vi "151126 thruster.vi"() -> ()   [LabVIEW 2015]
uses:
  <vilib>/MakerHub/LINX/Private/Type Defs/User Platform.ctl
  <vilib>/MakerHub/LINX/Private/Device/Type Defs/TCP Config.ctl
  <vilib>/MakerHub/LINX/Private/Type Defs/Interface.ctl
  <vilib>/MakerHub/LINX/Public/Sensors/Motion/Servo/Servo Open One Channel.vi
  <vilib>/MakerHub/Xbox-One-Controller/Public/Open First Controller.vi
  <vilib>/MakerHub/LINX/Public/Sensors/Motion/Servo/Servo Set Pulse Width One Channel.vi
  <vilib>/MakerHub/LINX/Public/Sensors/Motion/Servo/Servo Close One Channel.vi
  <vilib>/MakerHub/Xbox-One-Controller/LMH-Xbox-One-Controller.lvlib
  <vilib>/MakerHub/LINX/LMH-LINX.lvlib
  <vilib>/MakerHub/LINX/Public/Sensors/Motion/Servo/Servo.lvlib
  <vilib>/MakerHub/LINX/Private/Device/Device.lvlib
panel:
  in  "Stop Button":bool
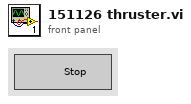
[diagram p1: front panel]
types:
  T1 = typedef "LMH-LINX.lvlib/Interface.ctl" = enum16{"Serial", "TCP"}
  T2 = typedef "LMH-LINX.lvlib/Device.lvlib/TCP Config.ctl" = cluster{"IP Address":string, "Port":u16}
  T3 = typedef "LMH-LINX.lvlib/User Platform.ctl" = enum16{"Default", "LINX", "myRIO"}
  T4 = typedef "LMH-LINX.lvlib/LINX Ref.ctl" = cluster{"Platform":T5, "Interface":T1, "LINX Device Config":T6}
  T5 = typedef "LMH-LINX.lvlib/Platform.ctl" = enum16{"LINX", "myRIO"}
  T6 = typedef "LMH-LINX.lvlib/Device.lvlib/LINX Device Config.ctl" = cluster{"Interface":T1, "COM Port":refnum<visa-resource-name>, "TCP Configuration":T2, "Device Family":u8, "Device ID":u8, "Device Name":string, "TCP Ref":refnum<k5>, "Channels":T7}
  T7 = typedef "LMH-LINX.lvlib/Channels.ctl" = cluster{"DI":u8[], "DO":u8[], "AI":u8[], "AO":u8[], "PWM":u8[], "QE":u8[], "UART":u8[], "I2C 2":u8[], "SPI":u8[], "CAN":u8[], "Servo":u8[], "AI Ref (V)":dbl, "AO Ref (V)":dbl, "AO Resolution (Bits)":u8}
  T8 = typedef "LMH-Xbox-One-Controller.lvlib/Xbox One Controller Ref.ctl" = cluster{"Controller Ref":refnum<k1>, "Event Refnum":refnum<event-registration>, "Worker Ref":refnum<vi>}
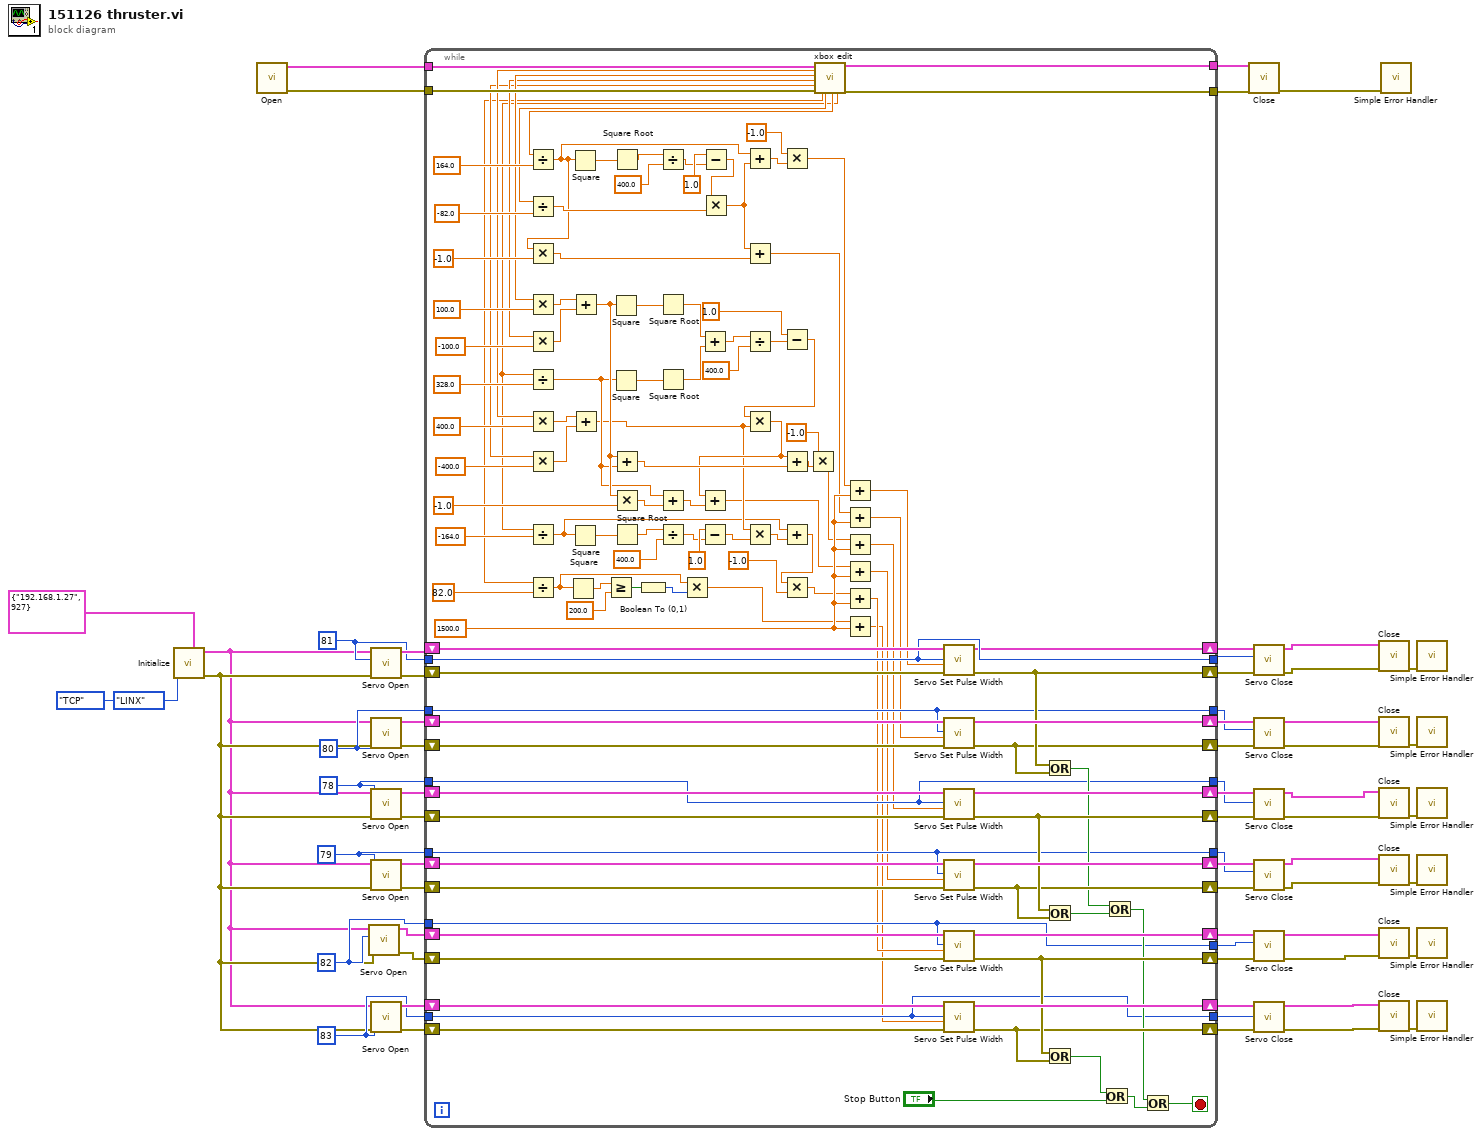
[diagram p0: block diagram]
diagram:
  w34 = u8 83 ("Servo Channel 6")
  w22 = u8 82 ("Servo Channel 5")
  w33 = u8 79 ("Servo Channel 4")
  w32 = u8 78 ("Servo Channel 3")
  w31 = u8 80 ("Servo Channel 2")
  w30 = u8 81 ("Servo Channel")
  n1 = call <vilib>:"Initialize.vi"("TCP Configuration"=T2 {"IP Address"="192.168.1.27", "Port"=927}, "Interface"=Interface."TCP", "Platform"=User_Platform."LINX") -> ("Error Out"=w3:errorcluster, "LINX Ref"=w2:T4)  [unwired: 6 in, 1 out]
  n2 = call-poly <vilib>:"Open.vi"() -> ("Error Out"=w36:errorcluster, "Xbox One Controller"=w38:T8)  [unwired: 9 in, 1 out]
  n3 = call-poly <vilib>:"Servo Open.vi"("Error In"=w3, "Servo Channel"=w22, "LINX Resource"=w2) -> ("Error Out"=w23:errorcluster, "LINX Resource"=w24:T4)  [unwired: 7 in]
  n4 = call-poly <vilib>:"Servo Open.vi"("Error In"=w3, "Servo Channel"=w30, "LINX Resource"=w2) -> ("Error Out"=w63:errorcluster, "LINX Resource"=w58:T4)  [unwired: 7 in]
  n5 = call-poly <vilib>:"Servo Open.vi"("Error In"=w3, "Servo Channel"=w31, "LINX Resource"=w2) -> ("Error Out"=w62:errorcluster, "LINX Resource"=w57:T4)  [unwired: 7 in]
  n6 = call-poly <vilib>:"Servo Open.vi"("Error In"=w3, "Servo Channel"=w32, "LINX Resource"=w2) -> ("Error Out"=w61:errorcluster, "LINX Resource"=w56:T4)  [unwired: 7 in]
  n7 = call-poly <vilib>:"Servo Open.vi"("Error In"=w3, "Servo Channel"=w33, "LINX Resource"=w2) -> ("Error Out"=w60:errorcluster, "LINX Resource"=w55:T4)  [unwired: 7 in]
  n8 = call-poly <vilib>:"Servo Open.vi"("Error In"=w3, "Servo Channel"=w34, "LINX Resource"=w2) -> ("Error Out"=w59:errorcluster, "LINX Resource"=w54:T4)  [unwired: 7 in]
  n9 = while {
    shift-right: [w66] -> w50
    shift-left: w58 -> [w180]
    shift-right: [w169] -> w44
    shift-left: w63 -> [w186]
    shift-right: [w174] -> w49
    shift-left: w57 -> [w179]
    shift-right: [w168] -> w43
    shift-left: w62 -> [w185]
    shift-right: [w173] -> w48
    shift-left: w56 -> [w178]
    shift-right: [w167] -> w42
    shift-left: w61 -> [w184]
    shift-right: [w172] -> w47
    shift-left: w55 -> [w177]
    shift-right: [w166] -> w41
    shift-left: w60 -> [w183]
    shift-right: [w171] -> w46
    shift-left: w24 -> [w176]
    shift-right: [w165] -> w40
    shift-left: w23 -> [w182]
    shift-right: [w170] -> w45
    shift-left: w54 -> [w175]
    shift-right: [w164] -> w39
    shift-left: w59 -> [w181]
    tunnel: w38 -> [w158]
    tunnel: [w157] -> w37
    tunnel: w36 -> [w156]
    tunnel: [w155] -> w35
    tunnel: w34 -> [w149]
    tunnel: w22 -> [w150]
    tunnel: w33 -> [w151]
    tunnel: w32 -> [w152]
    tunnel: w31 -> [w153]
    tunnel: w30 -> [w154]
    tunnel: [w154] -> w1
    tunnel: [w153] -> w29
    tunnel: [w152] -> w28
    tunnel: [w151] -> w27
    tunnel: [w150] -> w26
    tunnel: [w149] -> w25
    stop <- w65 stop-if-true
    w148 = 1500.0
    n10 = call "xbox edit.vi"("Xbox One Controller Ref"=w158, "Error In"=w156) -> ("Y"=w108:dbl, "B"=w125:dbl, "X"=w124:dbl, "A 2"=w107:dbl, "LS X"=w84:dbl, "LS Y"=w132:dbl, "RS X"=w142:dbl, "RS Y"=w79:dbl, "Xbox One Controller Ref"=w157:T8, "Error Out"=w155:errorcluster)  [unwired: 8 in]
    n11 = Divide(x=w142, y=164.0) -> (x/y=w131:dbl)
    n12 = Divide(x=w132, y=-82.0) -> (x/y=w140:dbl)
    n13 = Multiply(x=w131, y=-1.0) -> (x*y=w130:dbl)
    n14 = Multiply(x=w125, y=100.0) -> (x*y=w123:dbl)
    n15 = Multiply(x=w124, y=-100.0) -> (x*y=w122:dbl)
    n16 = Divide(x=w79, y=328.0) -> (x/y=w102:dbl)
    n17 = Multiply(x=w108, y=400.0) -> (x*y=w112:dbl)
    n18 = Multiply(x=w107, y=-400.0) -> (x*y=w111:dbl)
    n19 = Divide(x=w79, y=-164.0) -> (x/y=w88:dbl)
    n20 = Divide(x=w84, y=82.0) -> (x/y=w81:dbl)
    n21 = Square(x=w81) -> (x^2=w83:dbl)
    n22 = Square(x=w131) -> (x^2=w139:dbl)
    n23 = Square(x=w88) -> (x^2=w97:dbl)
    n24 = Add(x=w123, y=w122) -> (x+y=w103:dbl)
    n25 = Add(x=w112, y=w111) -> (x+y=w91:dbl)
    n26 = Greater Or Equal?(x=w83, y=200.0) -> (x >= y?=w87:bool)
    n27 = Square(x=w103) -> (x^2=w120:dbl)
    n28 = Square(x=w102) -> (x^2=w119:dbl)
    n29 = Square Root(x=w139) -> (sqrt(x)=w138:dbl)
    n30 = Add(x=w103, y=w102) -> (x+y=w105:dbl)
    n31 = Multiply(x=w103, y=-1.0) -> (x*y=w101:dbl)
    n32 = Square Root(x=w97) -> (sqrt(x)=w96:dbl)
    n33 = Boolean To (0,1)(Boolean=w87) -> (0, 1=w86:i16)
    n34 = Divide(x=w138, y=400.0) -> (x/y=w135:dbl)
    n35 = Square Root(x=w120) -> (sqrt(x)=w117:dbl)
    n36 = Square Root(x=w119) -> (sqrt(x)=w118:dbl)
    n37 = Add(x=w102, y=w101) -> (x+y=w100:dbl)
    n38 = Divide(x=w96, y=400.0) -> (x/y=w93:dbl)
    n39 = Multiply(x=w81, y=w86) -> (x*y=w80:dbl)
    n40 = Add(x=w117, y=w118) -> (x+y=w116:dbl)
    n41 = Subtract(x=1.0, y=w93) -> (x-y=w92:dbl)
    n42 = Subtract(x=1.0, y=w135) -> (x-y=w134:dbl)
    n43 = Multiply(x=w134, y=w140) -> (x*y=w129:dbl)
    n44 = Add(x=w131, y=w129) -> (x+y=w76:dbl)
    n45 = Add(x=w129, y=w130) -> (x+y=w128:dbl)
    n46 = Divide(x=w116, y=400.0) -> (x/y=w114:dbl)
    n47 = Multiply(x=w91, y=w92) -> (x*y=w89:dbl)
    n48 = Multiply(x=-1.0, y=w76) -> (x*y=w74:dbl)
    n49 = Subtract(x=1.0, y=w114) -> (x-y=w106:dbl)
    n50 = Multiply(x=w106, y=w91) -> (x*y=w99:dbl)
    n51 = Add(x=w99, y=w100) -> (x+y=w90:dbl)
    n52 = Add(x=w99, y=w105) -> (x+y=w73:dbl)
    n53 = Add(x=w88, y=w89) -> (x+y=w70:dbl)
    n54 = Multiply(x=w70, y=-1.0) -> (x*y=w68:dbl)
    n55 = Multiply(x=-1.0, y=w73) -> (x*y=w71:dbl)
    n56 = Add(x=w74, y=w148) -> (x+y=w144:dbl)
    n57 = Add(x=w128, y=w148) -> (x+y=w145:dbl)
    n58 = Add(x=w71, y=w148) -> (x+y=w146:dbl)
    n59 = Add(x=w90, y=w148) -> (x+y=w147:dbl)
    n60 = Add(x=w68, y=w148) -> (x+y=w78:dbl)
    n61 = Add(x=w80, y=w148) -> (x+y=w77:dbl)
    n62 = call-poly <vilib>:"Servo Set Pulse Width.vi"("Error In"=w186, "Pulse Width (uS)"=w144, "Servo Channel"=w154, "LINX Resource"=w180) -> ("Error Out"=w169:errorcluster, "LINX Resource"=w66:T4)  [unwired: 6 in]
    n63 = call-poly <vilib>:"Servo Set Pulse Width.vi"("Error In"=w185, "Pulse Width (uS)"=w145, "Servo Channel"=w153, "LINX Resource"=w179) -> ("Error Out"=w168:errorcluster, "LINX Resource"=w174:T4)  [unwired: 6 in]
    n64 = call-poly <vilib>:"Servo Set Pulse Width.vi"("Error In"=w184, "Pulse Width (uS)"=w146, "Servo Channel"=w152, "LINX Resource"=w178) -> ("Error Out"=w167:errorcluster, "LINX Resource"=w173:T4)  [unwired: 6 in]
    n65 = call-poly <vilib>:"Servo Set Pulse Width.vi"("Error In"=w183, "Pulse Width (uS)"=w147, "Servo Channel"=w151, "LINX Resource"=w177) -> ("Error Out"=w166:errorcluster, "LINX Resource"=w172:T4)  [unwired: 6 in]
    n66 = call-poly <vilib>:"Servo Set Pulse Width.vi"("Error In"=w182, "Pulse Width (uS)"=w78, "Servo Channel"=w150, "LINX Resource"=w176) -> ("Error Out"=w165:errorcluster, "LINX Resource"=w171:T4)  [unwired: 6 in]
    n67 = call-poly <vilib>:"Servo Set Pulse Width.vi"("Error In"=w181, "Pulse Width (uS)"=w77, "Servo Channel"=w149, "LINX Resource"=w175) -> ("Error Out"=w164:errorcluster, "LINX Resource"=w170:T4)  [unwired: 6 in]
    n68 = Or(x=w169, y=w168) -> (x .or. y?=w162:bool)
    n69 = Or(x=w167, y=w166) -> (x .or. y?=w163:bool)
    n70 = Or(x=w165, y=w164) -> (x .or. y?=w161:bool)
    n71 = Or(x=w161, y="Stop Button") -> (x .or. y?=w160:bool)
    n72 = Or(x=w162, y=w163) -> (x .or. y?=w159:bool)
    n73 = Or(x=w159, y=w160) -> (x .or. y?=w65:bool)
  }
  n74 = call <vilib>:"Close.vi"("Error In"=w35, "Xbox One Controller Ref"=w37) -> ("Error Out"=w64:errorcluster)  [unwired: 9 in]
  n75 = call-poly <vilib>:"Servo Close.vi"("Error In"=w44, "Servo Channel"=w1, "LINX Resource"=w50) -> ("Error Out"=w5:errorcluster, "LINX Resource"=w4:T4)  [unwired: 7 in]
  n76 = call-poly <vilib>:"Servo Close.vi"("Error In"=w43, "Servo Channel"=w29, "LINX Resource"=w49) -> ("Error Out"=w6:errorcluster, "LINX Resource"=w7:T4)  [unwired: 7 in]
  n77 = call-poly <vilib>:"Servo Close.vi"("Error In"=w42, "Servo Channel"=w28, "LINX Resource"=w48) -> ("Error Out"=w9:errorcluster, "LINX Resource"=w8:T4)  [unwired: 7 in]
  n78 = call-poly <vilib>:"Servo Close.vi"("Error In"=w41, "Servo Channel"=w27, "LINX Resource"=w47) -> ("Error Out"=w11:errorcluster, "LINX Resource"=w10:T4)  [unwired: 7 in]
  n79 = call-poly <vilib>:"Servo Close.vi"("Error In"=w40, "Servo Channel"=w26, "LINX Resource"=w46) -> ("Error Out"=w12:errorcluster, "LINX Resource"=w13:T4)  [unwired: 7 in]
  n80 = call-poly <vilib>:"Servo Close.vi"("Error In"=w39, "Servo Channel"=w25, "LINX Resource"=w45) -> ("Error Out"=w52:errorcluster, "LINX Resource"=w51:T4)  [unwired: 7 in]
  n81 = call <vilib>:"Close.vi"("Error In"=w5, "LINX Resource"=w4) -> ("Error Out"=w18:errorcluster)  [unwired: 8 in, 1 out]
  n82 = call <vilib>:"Close.vi"("Error In"=w6, "LINX Resource"=w7) -> ("Error Out"=w17:errorcluster)  [unwired: 8 in, 1 out]
  n83 = call <vilib>:"Close.vi"("Error In"=w9, "LINX Resource"=w8) -> ("Error Out"=w16:errorcluster)  [unwired: 8 in, 1 out]
  n84 = call <vilib>:"Close.vi"("Error In"=w11, "LINX Resource"=w10) -> ("Error Out"=w15:errorcluster)  [unwired: 8 in, 1 out]
  n85 = call <vilib>:"Close.vi"("Error In"=w12, "LINX Resource"=w13) -> ("Error Out"=w14:errorcluster)  [unwired: 8 in, 1 out]
  n86 = call <vilib>:"Close.vi"("Error In"=w52, "LINX Resource"=w51) -> ("Error Out"=w53:errorcluster)  [unwired: 8 in, 1 out]
  n87 = call <vilib>:"Simple Error Handler.vi"("error in (no error)"=w64) -> ()  [unwired: 4 in, 5 out]
  n88 = call <vilib>:"Simple Error Handler.vi"("error in (no error)"=w18) -> ()  [unwired: 4 in, 5 out]
  n89 = call <vilib>:"Simple Error Handler.vi"("error in (no error)"=w17) -> ()  [unwired: 4 in, 5 out]
  n90 = call <vilib>:"Simple Error Handler.vi"("error in (no error)"=w16) -> ()  [unwired: 4 in, 5 out]
  n91 = call <vilib>:"Simple Error Handler.vi"("error in (no error)"=w15) -> ()  [unwired: 4 in, 5 out]
  n92 = call <vilib>:"Simple Error Handler.vi"("error in (no error)"=w14) -> ()  [unwired: 4 in, 5 out]
  n93 = call <vilib>:"Simple Error Handler.vi"("error in (no error)"=w53) -> ()  [unwired: 4 in, 5 out]
